vi "Close.vi"(8 "error in (no error)":errorcluster, 11 "Huber Settings":T1) -> (0 "error out":errorcluster, 3 "Huber Settings":T1)   [LabVIEW 2018, in "Huber Ministat 230 TCU.lvlib"]
uses:
  Huber Ministat 230 TCU.lvlib
  Huber Settings.ctl
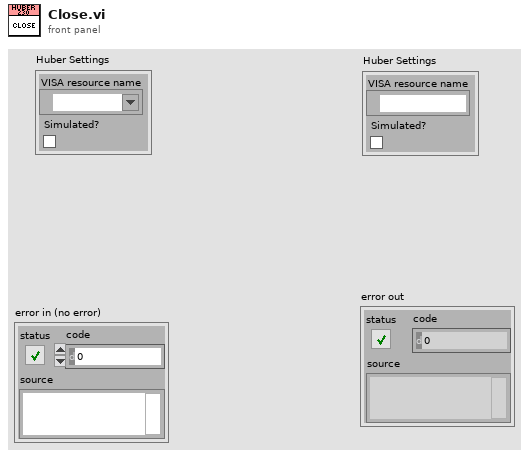
[diagram p1: front panel]
types:
  T1 = typedef "Huber Ministat 230 TCU.lvlib/Huber Settings.ctl" = cluster{"VISA resource name":refnum<visa-resource-name>, "Simulated?":bool}
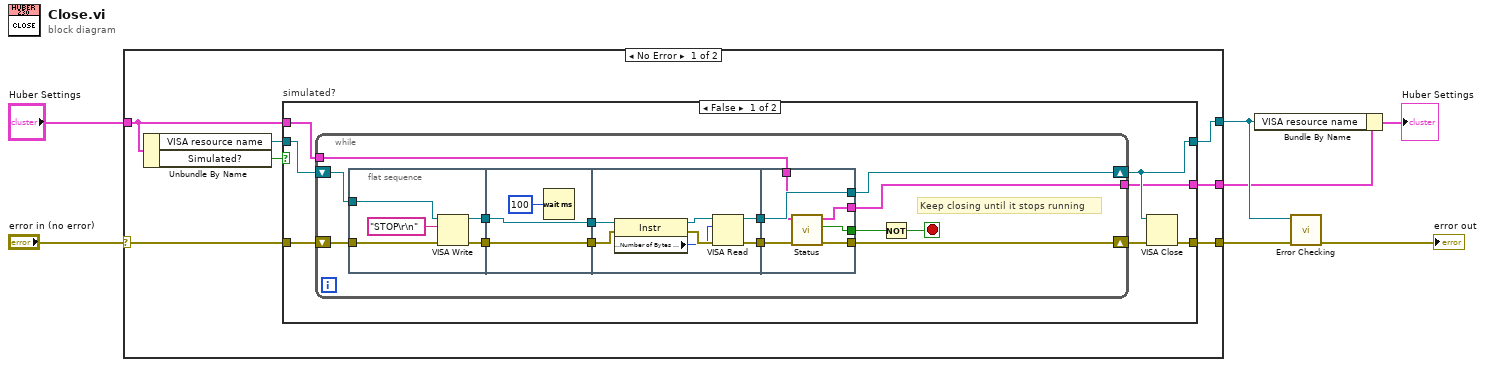
[diagram p0: block diagram]
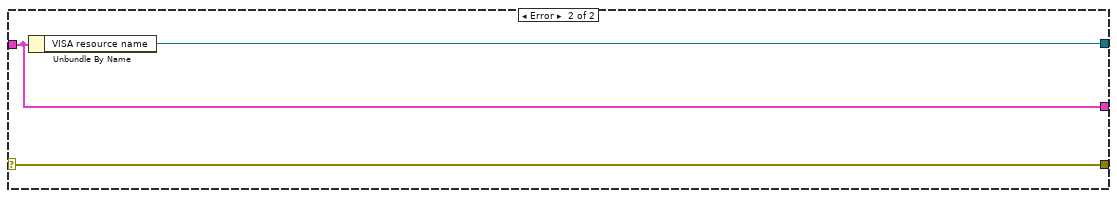
[diagram p3: hidden frame]
diagram:
  n1 = case shown="No Error" "error in (no error)" {
    selector: "error in (no error)" -> [w12 w62]
    tunnel: [w13 w62] -> w6
    tunnel: "Huber Settings" -> [w9 w60]
    tunnel: [w10 w61] -> w4
    tunnel: [w8 w60] -> w3
    frame No Error {
      n2 = Unbundle By Name(w9) -> ("VISA resource name"=w11:refnum<visa-resource-name>, "Simulated?"=w14:bool)
      n3 = case "simulated?" shown="False" w14 {
        tunnel: [w19 w59] -> w13
        tunnel: w11 -> [w18 w58]
        tunnel: w12 -> [w21 w59]
        tunnel: [w17 w58] -> w10
        tunnel: w9 -> [w16 w57]
        tunnel: [w15 w57] -> w8
        frame False {
          n4 = while {
            shift-right: [w28] -> w20
            shift-left: w21 -> [w29]
            shift-right: [w26] -> w17
            shift-left: w18 -> [w27]
            tunnel: w16 -> [w22]
            tunnel: [w23] -> w15
            stop <- w25 stop-if-true
            # "Keep closing until it stops running"
            n5 = flat-sequence {
              tunnel: [w37] -> w35
              tunnel: [w38] -> w34
              tunnel: w29 -> [w40]
              tunnel: w27 -> [w39]
              tunnel: w35 -> [w43]
              tunnel: [w43] -> w33
              tunnel: w34 -> [w42]
              tunnel: [w42] -> w32
              tunnel: w33 -> [w47]
              tunnel: w32 -> [w48]
              tunnel: [w50] -> w31
              tunnel: [w49] -> w30
              tunnel: [w56] -> w26
              tunnel: [w52] -> w28
              tunnel: w31 -> [w55]
              tunnel: w30 -> [w56]
              tunnel: [w51] -> w24
              tunnel: w22 -> [w54]
              tunnel: [w53] -> w23
              frame #0 {
                n6 = VISA Write(VISA resource name=w39, write buffer="STOP\r\n" ("string"), error in (no error)=w40) -> (VISA resource name out=w37:refnum<visa-resource-name>, error out=w38:errorcluster)  [unwired: 1 out]
              }
              frame #1 {
                n7 = Wait (ms)(milliseconds to wait=u32 100) -> ()  [unwired: 1 out]
              }
              frame #2 {
                n8 = property class="Instr"(reference=w47, error in=w48) -> (reference out=w46:refnum<visa-resource-name>, error out=w45:errorcluster, "Serial Settings:Number of Bytes at Serial Port"=w44:u32)
                n9 = VISA Read(VISA resource name=w46, byte count=w44, error in (no error)=w45) -> (VISA resource name out=w49:refnum<visa-resource-name>, error out=w50:errorcluster)  [unwired: 2 out]
              }
              frame #3 {
                n10 = call "Status.vi"("error in (no error)"=w55, "Huber Settings In"=w54) -> ("error out"=w52:errorcluster, "Running"=w51:bool, "Huber Settings Out"=w53:T1)  [unwired: 5 in, 2 out]
              }
            }
            n11 = Not(x=w24) -> (.not. x?=w25:bool)
          }
          n12 = VISA Close(VISA resource name=w17, error in (no error)=w20) -> (error out=w19:errorcluster)
        }
        frame True {
        }
      }
    }
    frame Error {
      n13 = Unbundle By Name(w60) -> ("VISA resource name"=w61:refnum<visa-resource-name>)
    }
  }
  n14 = Bundle By Name(cluster=w3, "VISA resource name"=w4) -> (→"Huber Settings":T1)
  n15 = call "Error Checking.vi"("error in (no error)"=w6, "VISA resource name"=w4) -> ("error out"=→"error out":errorcluster)  [unwired: 7 in, 2 out]
